vi "XYZ Queue.vi"() -> ()   [LabVIEW 2017]
uses:
  Program Files (x86)/National Instruments/LabVIEW 2017/examples/Instrument IO/Serial/support/Serial - Settings.ctl
  XY.ctl
  Z.ctl
  <vilib>/Instr/_visa.llb/VISA Configure Serial Port (Instr).vi
panel:
  in  "XY_Achse (Port 8)":refnum<visa-resource-name>="COM8"
  in  "XY Achse":T1={"Baudrate"=19200, "Datenbits"=8, "Parität"=enum."None", "Stoppbits"=10, "Ablaufsteuerung"=0} {"Ablaufsteuerung" items=["Keine"=0, "XON/XOFF"=1, "RTS/CTS"=2, "DTR/DSR"=4]; "Stoppbits" items=["1,0"=10, "1,5"=15, "2,0"=20]; "Datenbits" min=5 max=8 step=1; "Baudrate" items=["75"=75, "110"=110, "134"=134, "150"=150, "300"=300, "600"=600, "1200"=1200, "1800"=1800, "2400"=2400, "4800"=4800, "7200"=7200, "9600"=9600, "14400"=14400, "19200"=19200, "28800"=28800, "38400"=38400, "56000"=56000, "57600"=57600, "115200"=115200, "128000"=128000, "230400"=230400]}
  in  "Z_Achse (Port 9)":refnum<visa-resource-name>="COM9"
  in  "Z_Achse":T1={"Baudrate"=19200, "Datenbits"=8, "Parität"=enum."None", "Stoppbits"=10, "Ablaufsteuerung"=0} {"Ablaufsteuerung" items=["Keine"=0, "XON/XOFF"=1, "RTS/CTS"=2, "DTR/DSR"=4]; "Stoppbits" items=["1,0"=10, "1,5"=15, "2,0"=20]; "Datenbits" min=5 max=8 step=1; "Baudrate" items=["75"=75, "110"=110, "134"=134, "150"=150, "300"=300, "600"=600, "1200"=1200, "1800"=1800, "2400"=2400, "4800"=4800, "7200"=7200, "9600"=9600, "14400"=14400, "19200"=19200, "28800"=28800, "38400"=38400, "56000"=56000, "57600"=57600, "115200"=115200, "128000"=128000, "230400"=230400]}
  in  "Stopp":bool
  in  "XY_M_Trigger":bool
  in  "Z_M_Trigger":bool
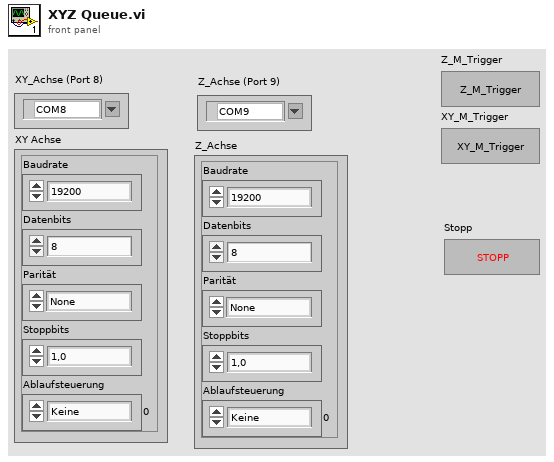
[diagram p1: front panel]
types:
  T1 = typedef "Serial - Settings.ctl" = cluster{"Baudrate":u32, "Datenbits":u16, "Parität":enum16{"None", "Odd", "Even", "Mark", "Space"}, "Stoppbits":u16, "Ablaufsteuerung":u16}
  T2 = typedef "Z.ctl" = enum16{"Z_Trigger", "Z_Stopp"}
  T3 = typedef "XY.ctl" = enum16{"XY_Trigger", "XY_Stopp"}
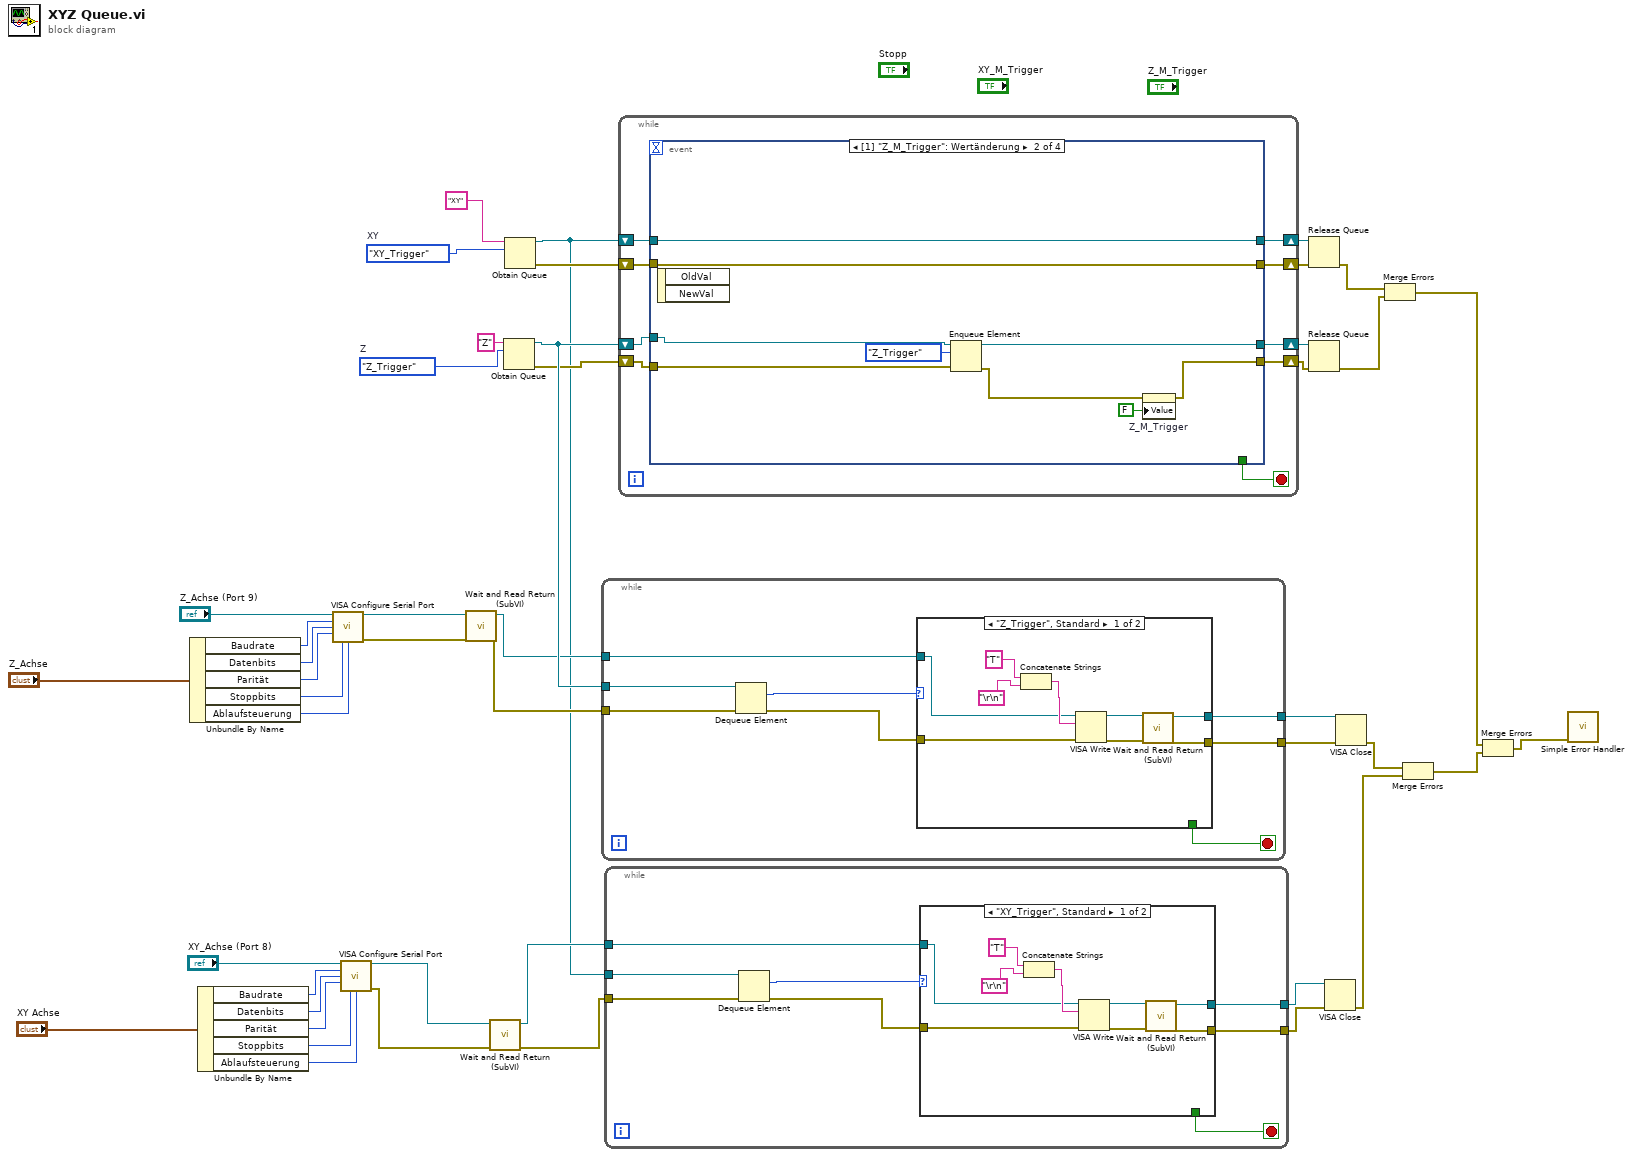
[diagram p0: block diagram]
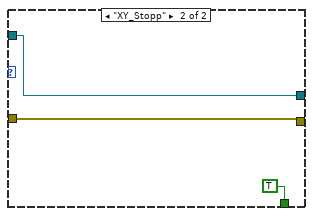
[diagram p2: hidden frame]
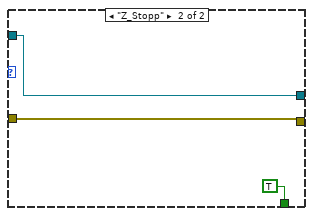
[diagram p3: hidden frame]
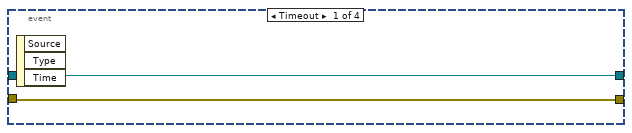
[diagram p4: hidden frame]
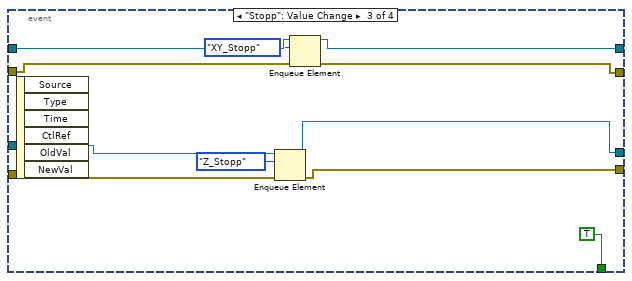
[diagram p5: hidden frame]
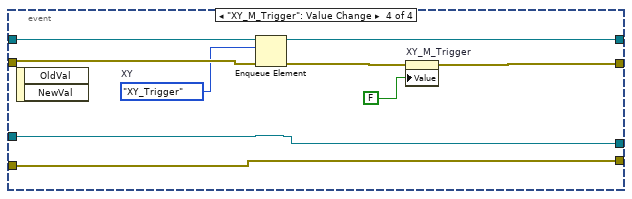
[diagram p6: hidden frame]
diagram:
  w37 = Z."Z_Trigger"  # Z
  w44 = XY."XY_Trigger"  # XY
  n1 = Unbundle By Name("Z_Achse") -> ("Baudrate"=w30:u32, "Datenbits"=w31:u16, "Parität"=w32:enum16{"None", "Odd", "Even", "Mark", "Space"}, "Stoppbits"=w33:u16, "Ablaufsteuerung"=w28:u16)
  n2 = Unbundle By Name("XY Achse") -> ("Baudrate"=w11:u32, "Datenbits"=w12:u16, "Parität"=w13:enum16{"None", "Odd", "Even", "Mark", "Space"}, "Stoppbits"=w14:u16, "Ablaufsteuerung"=w9:u16)
  n3 = call-poly "VISA Configure Serial Port"("VISA resource name"="Z_Achse (Port 9)", "baud rate (9600)"=w30, "data bits (8)"=w31, "parity (0:none)"=w32, "stop bits (10: 1 bit)"=w33, "flow control (0:none)"=w28) -> ("VISA resource name out"=w27:refnum<visa-resource-name>, "error out"=w23:errorcluster)  [unwired: 4 in, 4 out]
  n4 = call-poly "VISA Configure Serial Port"("VISA resource name"="XY_Achse (Port 8)", "baud rate (9600)"=w11, "data bits (8)"=w12, "parity (0:none)"=w13, "stop bits (10: 1 bit)"=w14, "flow control (0:none)"=w9) -> ("VISA resource name out"=w8:refnum<visa-resource-name>, "error out"=w7:errorcluster)  [unwired: 4 in, 4 out]
  n5 = call "Wait and Read Return (SubVI).vi"("Fehler (Eingang, kein Fehler)"=w23, "VISA-Referenz (Eingang)"=w27) -> ("Fehler (Ausgang)"=w20:errorcluster, "VISA-Referenz (Ausgang)"=w24:refnum<visa-resource-name>)  [unwired: 7 in, 1 out]
  n6 = call "Wait and Read Return (SubVI).vi"("Fehler (Eingang, kein Fehler)"=w7, "VISA-Referenz (Eingang)"=w8) -> ("Fehler (Ausgang)"=w5:errorcluster, "VISA-Referenz (Ausgang)"=w6:refnum<visa-resource-name>)  [unwired: 7 in, 1 out]
  n7 = Obtain Queue(name (unnamed)="Z" ("Name (unbenannt)"), element data type=w37) -> (queue out=w26:refnum<queue>, error out=w25:errorcluster)  [unwired: 3 in, 1 out]
  n8 = Obtain Queue(name (unnamed)="XY" ("Name (unbenannt)"), element data type=w44) -> (queue out=w4:refnum<queue>, error out=w43:errorcluster)  [unwired: 3 in, 1 out]
  n9 = while {
    tunnel: w26 -> [w53]
    tunnel: w24 -> [w51]
    tunnel: [w50] -> w22
    tunnel: [w48] -> w21
    tunnel: w20 -> [w46]
    stop <- w49 stop-if-true
    n10 = Dequeue Element(queue=w53, error in (no error)=w46) -> (element=w52:T2, error out=w47:errorcluster)  [unwired: 1 in, 2 out]
    n11 = case shown="\"Z_Trigger\", Standard" w52 {
      tunnel: w51 -> [w57 w65]
      tunnel: [w56 w65] -> w50
      tunnel: [_ TRUE] -> w49
      tunnel: [w55 w63] -> w48
      tunnel: w47 -> [w54 w63]
      frame "Z_Trigger", Default {
        n12 = Concatenate Strings("T" ("Schreibpuffer"), "\r\n") -> (w60:string)
        n13 = VISA Write(VISA resource name=w57, write buffer=w60, error in (no error)=w54) -> (VISA resource name out=w59:refnum<visa-resource-name>, error out=w58:errorcluster)  [unwired: 1 out]
        n14 = call "Wait and Read Return (SubVI).vi"("Fehler (Eingang, kein Fehler)"=w58, "VISA-Referenz (Eingang)"=w59) -> ("Fehler (Ausgang)"=w55:errorcluster, "VISA-Referenz (Ausgang)"=w56:refnum<visa-resource-name>)  [unwired: 7 in, 1 out]
      }
      frame "Z_Stopp" {
      }
    }
  }
  n15 = while {
    tunnel: w4 -> [w73]
    tunnel: w6 -> [w71]
    tunnel: [w70] -> w2
    tunnel: [w68] -> w3
    tunnel: w5 -> [w66]
    stop <- w69 stop-if-true
    n16 = Dequeue Element(queue=w73, error in (no error)=w66) -> (element=w72:T3, error out=w67:errorcluster)  [unwired: 1 in, 2 out]
    n17 = case shown="\"XY_Trigger\", Standard" w72 {
      tunnel: w71 -> [w77 w85]
      tunnel: [w76 w85] -> w70
      tunnel: [_ TRUE] -> w69
      tunnel: [w75 w83] -> w68
      tunnel: w67 -> [w74 w83]
      frame "XY_Trigger", Default {
        n18 = Concatenate Strings("T" ("Schreibpuffer"), "\r\n") -> (w80:string)
        n19 = VISA Write(VISA resource name=w77, write buffer=w80, error in (no error)=w74) -> (VISA resource name out=w79:refnum<visa-resource-name>, error out=w78:errorcluster)  [unwired: 1 out]
        n20 = call "Wait and Read Return (SubVI).vi"("Fehler (Eingang, kein Fehler)"=w78, "VISA-Referenz (Eingang)"=w79) -> ("Fehler (Ausgang)"=w75:errorcluster, "VISA-Referenz (Ausgang)"=w76:refnum<visa-resource-name>)  [unwired: 7 in, 1 out]
      }
      frame "XY_Stopp" {
      }
    }
  }
  n21 = while {
    shift-right: [w92] -> w42
    shift-left: w4 -> [w94]
    shift-right: [w91] -> w41
    shift-left: w43 -> [w93]
    shift-right: [w88] -> w39
    shift-left: w26 -> [w90]
    shift-right: [w87] -> w38
    shift-left: w25 -> [w89]
    stop <- w86 stop-if-true
    n22 = event shown="[1] \"Z_M_Trigger\": Wertänderung" {
      selector: _ -> [_ _ _ _]
      dyn-events: _ -> [_ _ _ _]
      timeout: _ -> [_ _ _ _]
      tunnel: w94 -> [w96 w103 w112 w125]
      tunnel: w93 -> [w95 w102 w113 w124]
      tunnel: [w96 w103 w111 w123] -> w92
      tunnel: [w95 w102 w110 w120] -> w91
      tunnel: w90 -> [_ w104 w115 w118]
      tunnel: w89 -> [_ w105 w114 w117]
      tunnel: [_ w101 w116 w118] -> w88
      tunnel: [_ w98 w106 w117] -> w87
      tunnel: [_ _ TRUE _] -> w86
      event Timeout {
        n23 = event-data() -> ()  [unwired: 1 in, 3 out]
      }
      event "Z_M_Trigger": Value Change {
        n24 = event-data() -> ()  [unwired: 1 in, 2 out]
        n25 = Enqueue Element(queue=w104, element=Z."Z_Trigger" ("Element"), error in (no error)=w105) -> (queue out=w101:refnum<queue>, error out=w99:errorcluster)  [unwired: 1 in, 1 out]
        n26 = property on="Z_M_Trigger" class="Bool. (strikt)"(error in=w99, "Value"=FALSE ("Z_M_Trigger")) -> (error out=w98:errorcluster)  [unwired: 1 in, 1 out]
      }
      event "Stopp": Value Change {
        n27 = event-data() -> ()  [unwired: 1 in, 6 out]
        n28 = Enqueue Element(queue=w115, element=Z."Z_Stopp" ("Element"), error in (no error)=w114) -> (queue out=w116:refnum<queue>, error out=w106:errorcluster)  [unwired: 1 in, 1 out]
        n29 = Enqueue Element(queue=w112, element=XY."XY_Stopp" ("Element"), error in (no error)=w113) -> (queue out=w111:refnum<queue>, error out=w110:errorcluster)  [unwired: 1 in, 1 out]
      }
      event "XY_M_Trigger": Value Change {
        w122 = XY."XY_Trigger"  # XY
        n30 = event-data() -> ()  [unwired: 1 in, 2 out]
        n31 = Enqueue Element(queue=w125, element=w122, error in (no error)=w124) -> (queue out=w123:refnum<queue>, error out=w121:errorcluster)  [unwired: 1 in, 1 out]
        n32 = property on="XY_M_Trigger" class="Bool. (strikt)"(error in=w121, "Value"=FALSE ("XY_M_Trigger")) -> (error out=w120:errorcluster)  [unwired: 1 in, 1 out]
      }
    }
  }
  n33 = Release Queue(queue=w42, error in (no error)=w41) -> (error out=w36:errorcluster)  [unwired: 1 in, 2 out]
  n34 = Release Queue(queue=w39, error in (no error)=w38) -> (error out=w35:errorcluster)  [unwired: 1 in, 2 out]
  n35 = VISA Close(VISA resource name=w2, error in (no error)=w3) -> (error out=w1:errorcluster)
  n36 = VISA Close(VISA resource name=w22, error in (no error)=w21) -> (error out=w19:errorcluster)
  n37 = Merge Errors(w36, w35) -> (w18:errorcluster)
  n38 = Merge Errors(w19, w1) -> (w17:errorcluster)
  n39 = Merge Errors(w18, w17) -> (w16:errorcluster)
  n40 = call <vilib>:"Simple Error Handler.vi"("error in (no error)"=w16) -> ()  [unwired: 4 in, 5 out]
